vi "LVUSBRH2_Measurement_SUB_SelectComPort_Panel.vi"(11 "VISA rsrc in":refnum<visa-resource-name> caption="COM port in") -> (1 "Cancel?":bool, 3 "VISA rsrc out":refnum<visa-resource-name> caption="COM port out")   [LabVIEW 2020]
uses:
  <vilib>/Instr/_visa.llb/VISA Configure Serial Port (Instr).vi
panel:
  in  "Btn CommTest":bool
  in  "Btn Cancel":bool
  in  "Btn OK":bool
  in  "VISA rsrc":refnum<visa-resource-name> caption="COM port"
  # "Select COM port for USBRH2"
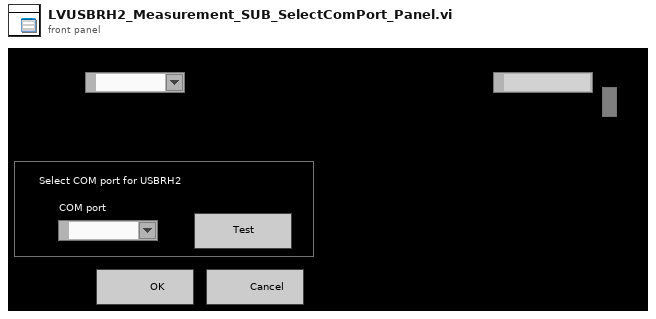
[diagram p1: front panel]
types:
  T1 = enum32{"Invalid", "Default", "Floating", "Floating/Auto-Hide", "Modal"}
  T2 = enum8{"Enabled", "Disabled", "Disabled and Grayed Out"}
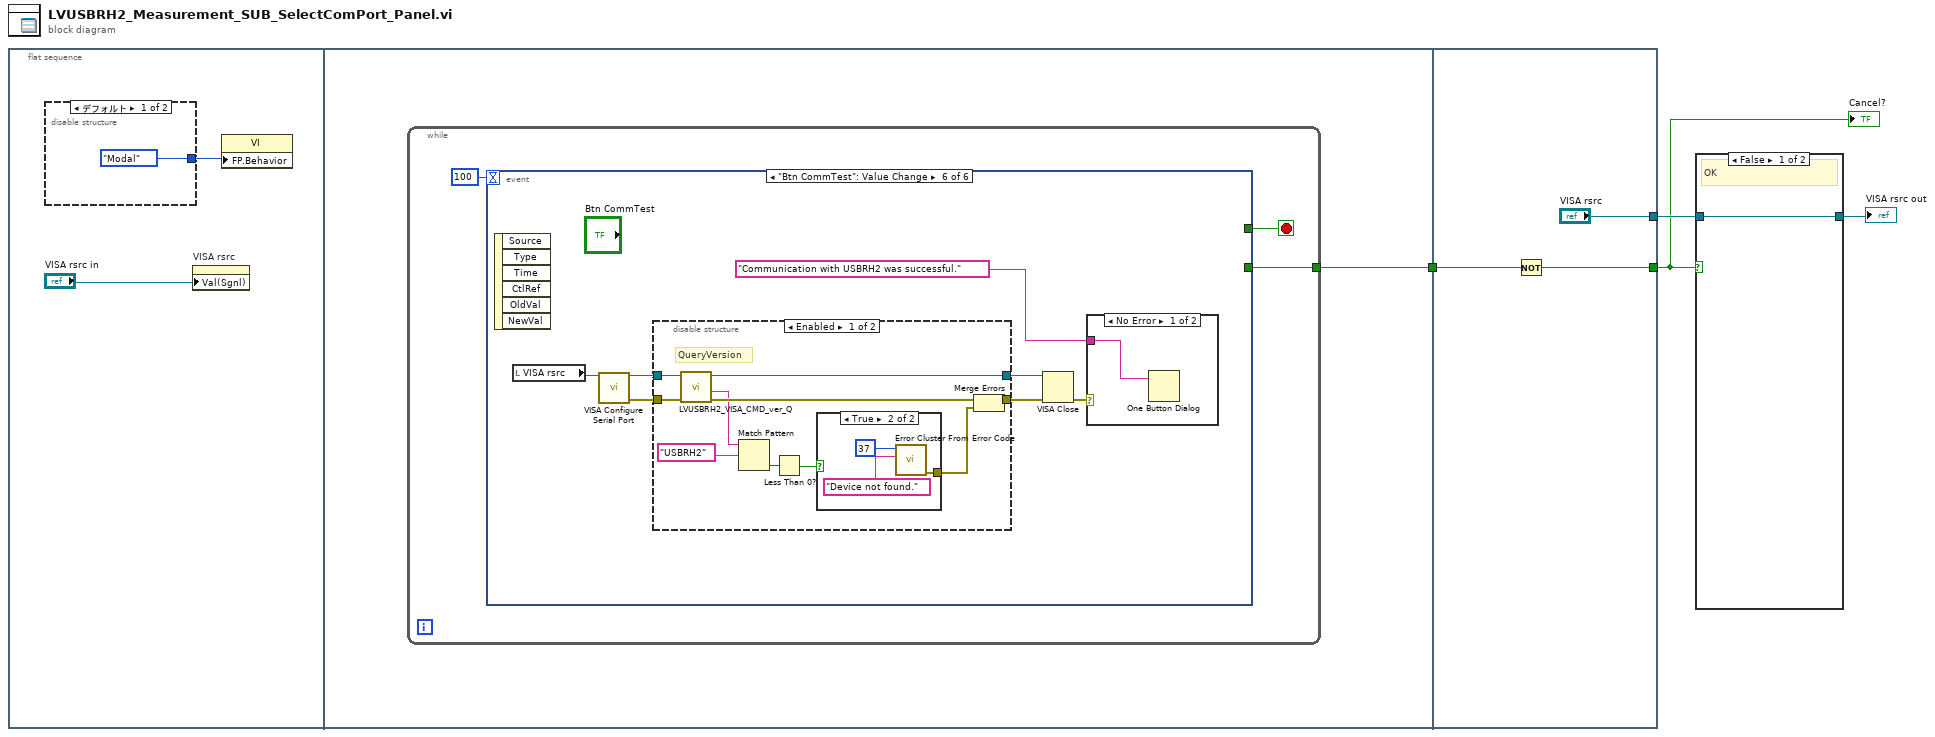
[diagram p0: block diagram]
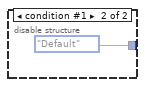
[diagram p3: hidden frame]
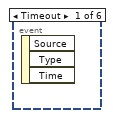
[diagram p4: hidden frame]
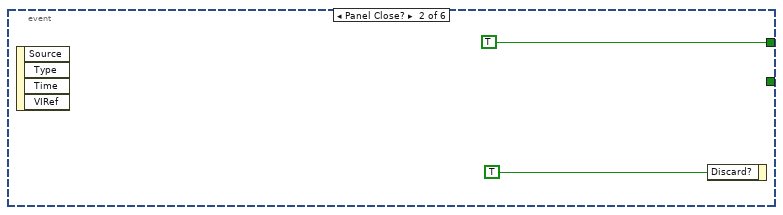
[diagram p5: hidden frame]
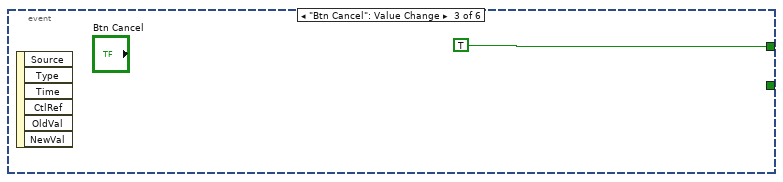
[diagram p6: hidden frame]
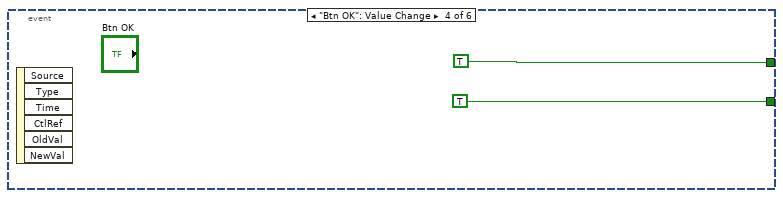
[diagram p7: hidden frame]
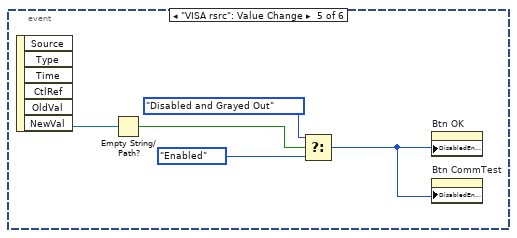
[diagram p8: hidden frame]
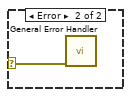
[diagram p11: hidden frame]
diagram:
  n1 = flat-sequence {
    tunnel: [w9] -> w4
    tunnel: [w47] -> w1
    tunnel: w4 -> [w49]
    tunnel: ["VISA rsrc"] -> w3
    frame #0 {
      n2 = disable-structure shown="デフォルト" {
        disable-tunnel: [T1."Modal" ("フロントパネルウィンドウ:動作") T1."Default" ("フロントパネルウィンドウ:動作")] -> w5
        frame condition #0 (active) {
        }
        frame condition #1 {
        }
      }
      n3 = property on="VISA rsrc" class="VISAName"("Val(Sgnl)"="VISA rsrc in") -> ()  [unwired: 2 in, 2 out]
      n4 = property class="VI"("FP.Behavior"=w5) -> ()  [unwired: 2 in, 2 out]
    }
    frame #1 {
      n5 = while {
        tunnel: [w10] -> w9
        stop <- w11 stop-if-true
        n6 = event shown="[5] \"Btn CommTest\": Value Change" {
          selector: _ -> [_ _ _ _ _ _]
          dyn-events: _ -> [_ _ _ _ _ _]
          timeout: 100 -> [_ _ _ _ _ _]
          tunnel: [_ TRUE TRUE TRUE _ _] -> w11
          tunnel: [_ _ _ TRUE _ _] -> w10
          event Timeout {
            n7 = event-data() -> ()  [unwired: 1 in, 3 out]
          }
          event Panel Close? {
            n8 = event-data() -> ()  [unwired: 1 in, 4 out]
            n9 = event-data("Discard?"=TRUE ("破棄?")) -> ()  [unwired: 1 in, 1 out]
          }
          event "Btn Cancel": Value Change {
            n10 = event-data() -> ()  [unwired: 1 in, 6 out]
          }
          event "Btn OK": Value Change {
            n11 = event-data() -> ()  [unwired: 1 in, 6 out]
          }
          event "VISA rsrc": Value Change {
            n12 = event-data() -> ("NewVal"=w22:refnum<visa-resource-name>)  [unwired: 1 in, 5 out]
            n13 = Empty String/Path?(string/path=w22) -> (empty?=w20:bool)
            n14 = Select(t=T2."Disabled and Grayed Out" ("無効"), s=w20, f=T2."Enabled" ("無効")) -> (s? t:f=w18:T2)
            n15 = property on="Btn OK" class="Bool"("DisabledEnum"=w18) -> ()  [unwired: 2 in, 2 out]
            n16 = property on="Btn CommTest" class="Bool"("DisabledEnum"=w18) -> ()  [unwired: 2 in, 2 out]
          }
          event "Btn CommTest": Value Change {
            n17 = event-data() -> ()  [unwired: 1 in, 6 out]
            n18 = local read "VISA rsrc"() -> (w29:refnum<visa-resource-name>)
            n19 = call-poly "VISA Configure Serial Port"("VISA resource name"=w29) -> ("VISA resource name out"=w26:refnum<visa-resource-name>, "error out"=w24:errorcluster)  [unwired: 13 in]
            n20 = disable-structure shown="Enabled" {
              disable-tunnel: w26 -> [w39 w44]
              disable-tunnel: [w38 w44] -> w25
              disable-tunnel: w24 -> [w37 w43]
              disable-tunnel: [w31 w43] -> w23
              frame Enabled {
                # "QueryVersion"
                n21 = call "LVUSBRH2_VISA_CMD_ver_Q.vi"("error in (no error)"=w37, "VISA rssc"=w39) -> ("error out"=w36:errorcluster, "recv string"=w34:string, "VISA rssc out"=w38:refnum<visa-resource-name>)  [unwired: 7 in]
                n22 = Match Pattern(string=w34, regular expression="USBRH2") -> (offset past match=w33:i32)  [unwired: 1 in, 3 out]
                n23 = Less Than 0?(x=w33) -> (x < 0?=w32:bool)
                n24 = case shown="True" w32 {
                  tunnel: [_ w40] -> w30
                  frame False {
                  }
                  frame True {
                    n25 = call <vilib>:"Error Cluster From Error Code.vi"("error message (\"\")"="Device not found." ("error message (\"\")"), "error code (0)"=37) -> ("error out"=w40:errorcluster)  [unwired: 7 in]
                  }
                }
                n26 = Merge Errors(w36, w30) -> (w31:errorcluster)
              }
              frame Disabled {
              }
            }
            n27 = VISA Close(VISA resource name=w25, error in (no error)=w23) -> (error out=w28:errorcluster)
            n28 = case shown="No Error" w28 {
              selector: w28 -> [_ w46]
              tunnel: "Communication with USBRH2 was successful." ("メッセージ") -> [w45 _]
              frame No Error {
                n29 = One Button Dialog(message=w45) -> ()  [unwired: 1 in, 1 out]
              }
              frame Error {
                n30 = call <vilib>:"General Error Handler.vi"("error in (no error)"=w46) -> ()  [unwired: 10 in, 5 out]
              }
            }
          }
        }
      }
    }
    frame #2 {
      n31 = Not(x=w49) -> (.not. x?=w47:bool)
    }
  }
  n32 = case shown="False" w1 {
    tunnel: [w50 _] -> w2
    tunnel: w3 -> [w50 _]
    frame False {
      # "OK"
    }
    frame True {
      # "Cancel"
    }
  }
  "VISA rsrc out" <- w2
  "Cancel?" <- w1
